vi "SeqMgr.Data 1D Load from File.vi"(8 "error in (no error)":errorcluster, 11 "Args":string[](array[string])) -> (0 "error out":errorcluster, 1 "Max Indices":string[][](array[string]), 2 "Data":string[](array[string]), 3 "Name":string)   [LabVIEW 2024, in "EQMF.lvlib" / "SeqMgr.lvlib"]
uses:
  SeqMgr.lvlib
  <vilib>/Utility/error.llb/Trim Whitespace One-Sided.vi
panel:
  # "Data1DLoadFromFile(VarName, MaxIndex, Path,[Delimiter,ExcludeHeaderCnt])"
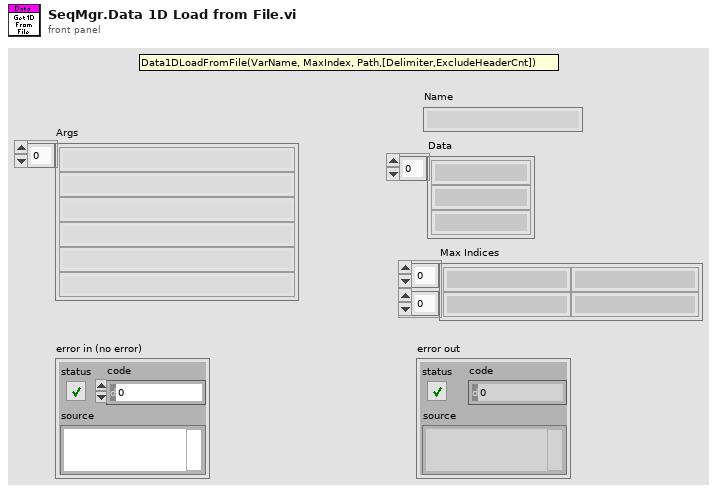
[diagram p1: front panel]
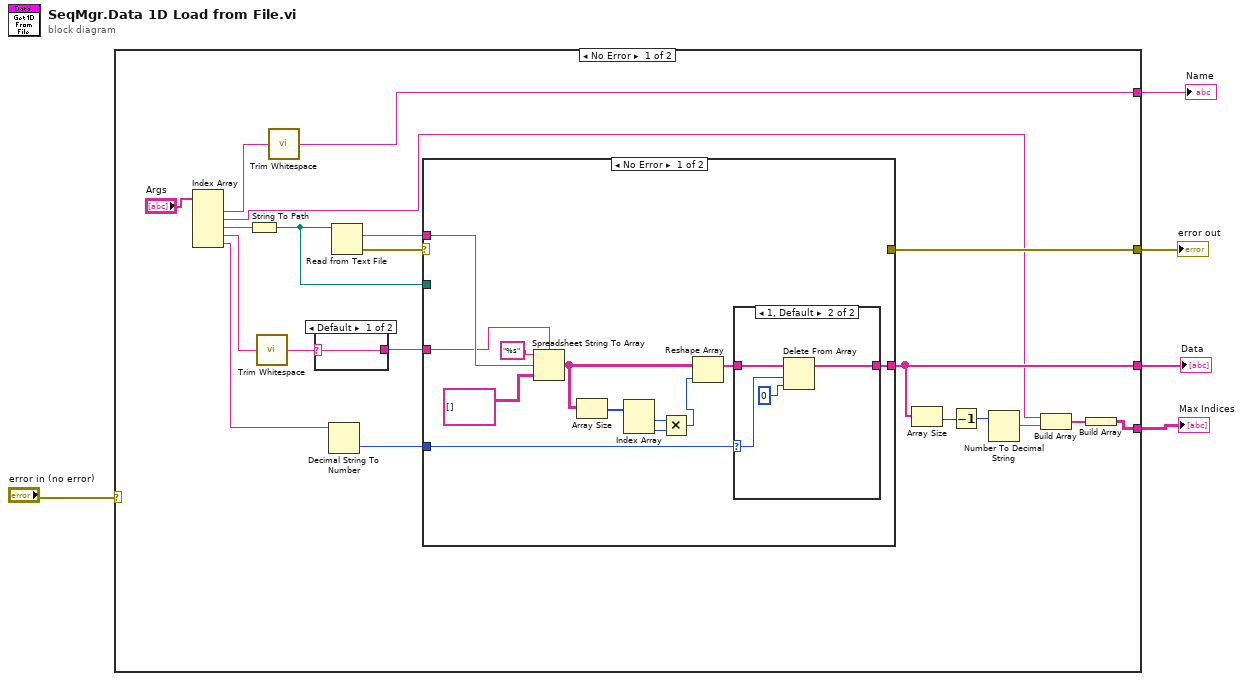
[diagram p0: block diagram]
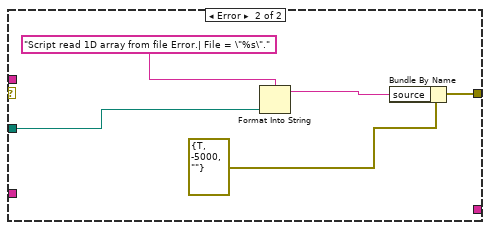
[diagram p3: hidden frame]
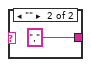
[diagram p4: hidden frame]
diagram:
  n1 = case shown="No Error" "error in (no error)" {
    selector: "error in (no error)" -> [_ w50]
    tunnel: [w18 _] -> w5
    tunnel: [w13 _] -> w4
    tunnel: [w15 w50] -> w3
    tunnel: [w6 _] -> w1
    frame No Error {
      n2 = Index Array(array="Args") -> (element #1=w9:string, element #2=w8:string, element #3=w25:string, element #4=w23:string, element #5=w20:string)  [unwired: 5 in]
      n3 = String To Path(string=w25) -> (path=w14:path)
      n4 = call <vilib>:"Trim Whitespace.vi"("string"=w23) -> ("trimmed string"=w22:string)  [unwired: 1 in]
      n5 = call <vilib>:"Trim Whitespace.vi"("string"=w9) -> ("trimmed string"=w18:string)  [unwired: 1 in]
      n6 = case shown="Default" w22 {
        selector: w22 -> [w48 _]
        tunnel: [w48 ","] -> w21
        frame Default {
        }
        frame "" {
        }
      }
      n7 = Decimal String To Number(string=w20) -> (number=w17:i32)  [unwired: 2 in, 1 out]
      n8 = Read from Text File(file (use dialog)=w14) -> (text=w24:string, error out=w16:errorcluster)  [unwired: 3 in, 2 out]
      n9 = case shown="No Error" w16 {
        tunnel: w24 -> [w37 _]
        tunnel: w21 -> [w35 _]
        tunnel: w17 -> [w33 _]
        tunnel: [w32 _] -> w13
        tunnel: [_ w43] -> w15
        tunnel: w14 -> [_ w46]
        frame No Error {
          n10 = Spreadsheet String To Array(delimiter (Tab)=w35, format string="%s", spreadsheet string=w37, array type (2D Dbl)=string[][] [] ("Data")) -> (array=w30:string[][])
          n11 = Array Size(array=w30) -> (size(s)=w29:i32[])
          n12 = Index Array(array=w29) -> (element #1=w28:i32, element #2=w27:i32)  [unwired: 2 in]
          n13 = Multiply(x=w28, y=w27) -> (x*y=w26:i32)
          n14 = Reshape Array(w30, w26) -> (w31:string[])
          n15 = case shown="1, Default" w33 {
            selector: w33 -> [_ w41]
            tunnel: w31 -> [w38 w42]
            tunnel: [w38 w40] -> w32
            frame 0 {
            }
            frame 1, Default {
              n16 = Delete From Array(array=w42, length=w41, index=0 ("index (row)")) -> (array with subset deleted=w40:string[])  [unwired: 1 out]
            }
          }
        }
        frame Error {
          n17 = Format Into String(format string="Script read 1D array from file Error.| File = \"%s\".", w46) -> (resulting string=w44:string)  [unwired: 2 in, 1 out]
          n18 = Bundle By Name(cluster=errorcluster {"status"=TRUE, "code"=-5000, "source"=""} ("error constant"), "source"=w44) -> (w43:errorcluster)
        }
      }
      n19 = Array Size(array=w13) -> (size(s)=w10:i32)
      n20 = Decrement(x=w10) -> (x-1=w11:i32)
      n21 = Number To Decimal String(number=w11) -> (decimal integer string=w12:string)  [unwired: 1 in]
      n22 = Build Array(w8, w12) -> (w7:string[])
      n23 = Build Array(w7) -> (w6:string[][])
    }
    frame Error {
    }
  }
  "Data" <- w4
  "error out" <- w3
  "Name" <- w5
  "Max Indices" <- w1
